vi "equ (SubVI).vi"(0 "Entrada":waveform(dbl), 1 "Bajos":dbl, 2 "Medios":dbl, 3 "Agudos":dbl, 4 "Indice de Bloque":i32) -> (5 "Salida":waveform(dbl))   [LabVIEW 2013]
uses:
  <vilib>/Analysis/NI_AALBase.lvlib
  <vilib>/Analysis/3filter.llb/Chebyshev Filter (DBL).vi
  <vilib>/Analysis/3filter.llb/Filter Passband Type.ctl
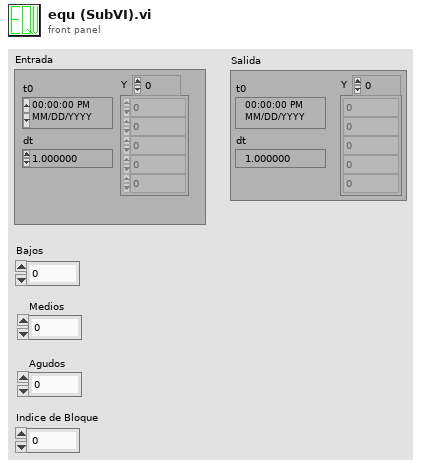
[diagram p1: front panel]
types:
  T1 = typedef "NI_AALBase.lvlib/Filter Passband Type.ctl" = enum32{"Lowpass", "Highpass", "Bandpass", "Bandstop"}
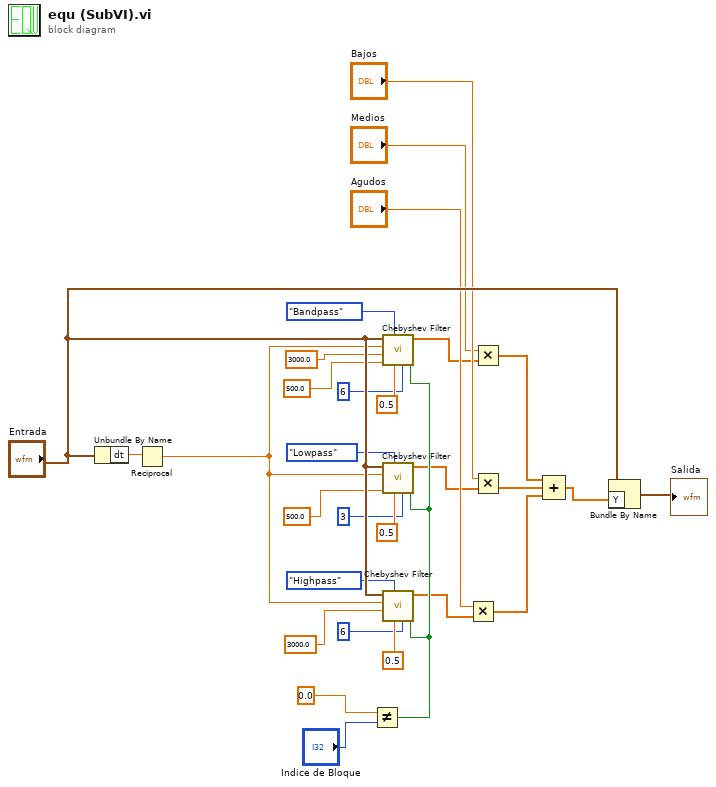
[diagram p0: block diagram]
diagram:
  n1 = Unbundle By Name("Entrada") -> ("dt"=w14:dbl)
  n2 = Reciprocal(x=w14) -> (1/x=w15:dbl)
  n3 = Not Equal?(x=0.0, y="Indice de Bloque") -> (x != y?=w28:bool)
  n4 = call-poly <vilib>:"Chebyshev Filter.vi"("init/cont (init:F)"=w28, "order"=6, "ripple(dB)"=0.5, "filter type"=Filter_Passband_Type."Bandpass", "low cutoff freq: fl"=500.0, "high cutoff freq: fh"=3000.0, "sampling freq: fs"=w15, "X"="Entrada") -> ("Filtered X"=w17:dbl[])  [unwired: 2 in, 1 out]
  n5 = call-poly <vilib>:"Chebyshev Filter.vi"("init/cont (init:F)"=w28, "order"=3, "ripple(dB)"=0.5, "filter type"=Filter_Passband_Type."Lowpass", "low cutoff freq: fl"=500.0, "sampling freq: fs"=w15, "X"="Entrada") -> ("Filtered X"=w19:dbl[])  [unwired: 3 in, 1 out]
  n6 = call-poly <vilib>:"Chebyshev Filter.vi"("init/cont (init:F)"=w28, "order"=6, "ripple(dB)"=0.5, "filter type"=Filter_Passband_Type."Highpass", "high cutoff freq: fh"=3000.0, "sampling freq: fs"=w15, "X"="Entrada") -> ("Filtered X"=w21:dbl[])  [unwired: 3 in, 1 out]
  n7 = Multiply(x="Agudos", y=w21) -> (x*y=w24:dbl[])
  n8 = Multiply(x="Medios", y=w17) -> (x*y=w22:dbl[])
  n9 = Multiply(x="Bajos", y=w19) -> (x*y=w23:dbl[])
  n10 = Compound Arithmetic op=ADD(w22, w23, w24) -> (w25:dbl[])
  n11 = Bundle By Name(cluster="Entrada", "Y"=w25) -> (→"Salida":waveform(dbl))
